vi "Run.vi"(8 "error in (no error)":errorcluster caption="entrée d'erreur (pas d'erreur)", 9 "Y":string[][](array[string]), 10 "X":string[][](array[string]), 11 "Laplacian_kernel.lvclass":refnum<class "Laplacian_kernel.lvclass">) -> (0 "error out":errorcluster caption="sortie d'erreur", 2 "Data":T1, 3 "Laplacian_kernel.lvclass":refnum<class "Laplacian_kernel.lvclass">)   [LabVIEW 2020, in "Laplacian_kernel.lvclass"]
doc: "Returns : \n\n- kernel_matrix : array of shape (n_samples_X, n_samples_Y)"
uses:
  Laplacian_kernel.lvclass
  Laplacian_kernel.lvclass/Laplacian_kernel.ctl
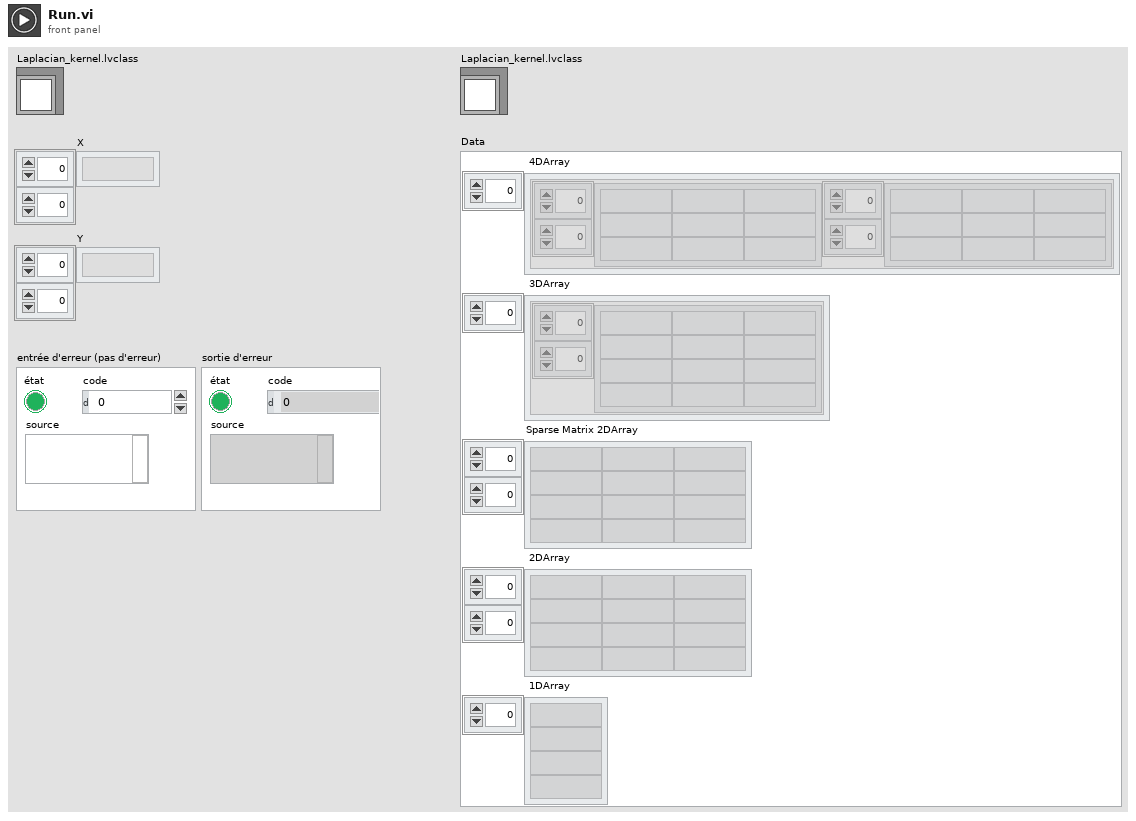
[diagram p1: front panel]
types:
  T1 = cluster{" 4DArray":cluster{"1":string[][], "2":string[][]}[], " 3DArray":cluster{"Tableau":string[][]}[], "Sparse Matrix 2DArray":string[][], " 2DArray":string[][], " 1DArray":string[]}
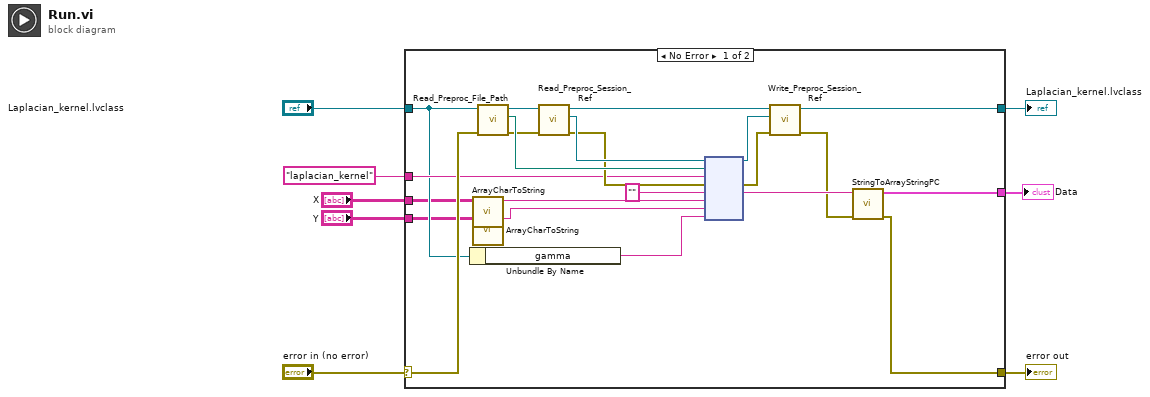
[diagram p0: block diagram]
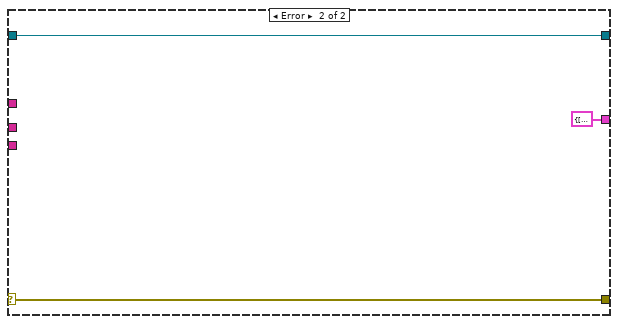
[diagram p2: hidden frame]
diagram:
  n1 = case shown="No Error" "error in (no error)" {
    selector: "error in (no error)" -> [w21 w33]
    tunnel: [w9 w33] -> w7
    tunnel: [w13 w32] -> w5
    tunnel: "Laplacian_kernel.lvclass" -> [w19 w32]
    tunnel: "laplacian_kernel" ("Fonction") -> [w20 _]
    tunnel: "X" -> [w17 _]
    tunnel: "Y" -> [w14 _]
    tunnel: [w10 T1 {" 4DArray"=[], " 3DArray"=[], "Sparse Matrix 2DArray"=[], " 2DArray"=[], " 1DArray"=[]} ("Data")] -> w1
    frame No Error {
      n2 = Unbundle By Name(w19) -> ("gamma"=w18:string)
      n3 = call "ArrayCharToString.vi"("TAB"=w17) -> ("Instruction"=w16:string)  [unwired: 10 in]
      n4 = call "ArrayCharToString.vi"("TAB"=w14) -> ("Instruction"=w15:string)  [unwired: 10 in]
      n5 = call-dynamic "Read_Preproc_File_Path.vi"("error in (no error)"=w21, "Python in"=w19) -> ("error out"=w25:errorcluster, "File_Path"=w28:path, "Python out"=w30:refnum<class "Laplacian_kernel.lvclass">)  [unwired: 7 in]
      n6 = call-dynamic "Read_Preproc_Session_Ref.vi"("error in (no error)"=w25, "Python in"=w30) -> ("error out"=w26:errorcluster, "Session_ref"=w27:refnum<k35>, "Python out"=w29:refnum<class "Laplacian_kernel.lvclass">)  [unwired: 7 in]
      n7 = node(w27, w28, w20, w26, "", w16, w15, w18) -> (w22:refnum<k35>, w24:errorcluster, w12:string)  [unwired: 3 in, 2 out]
      n8 = call-dynamic "Write_Preproc_Session_Ref.vi"("error in (no error)"=w24, "Session_ref"=w22, "Python in"=w29) -> ("error out"=w11:errorcluster, "Python out"=w13:refnum<class "Laplacian_kernel.lvclass">)  [unwired: 7 in]
      n9 = call "StringToArrayStringPC.vi"("sortie d'erreur"=w11, "Return value"=w12) -> ("sortie d'erreur"=w9:errorcluster, "Data"=w10:T1)  [unwired: 8 in]
    }
    frame Error {
    }
  }
  "error out" <- w7
  "Laplacian_kernel.lvclass" <- w5
  "Data" <- w1
